vi "Test MPU6050 1.vi"(8 "Error In":errorcluster) -> (0 "error out":errorcluster)   [LabVIEW 2014]
uses:
  <vilib>/LabVIEW Universal Transcriptor/Arduino MPU6050 Library/Arduino MPU6050.lvlib
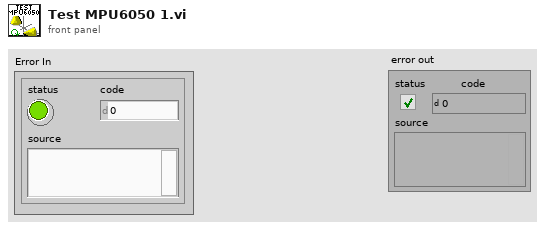
[diagram p1: front panel]
types:
  T1 = enum16{"MPU6050_SCALE_250DPS", "MPU6050_SCALE_500DPS", "MPU6050_SCALE_1000DPS", "MPU6050_SCALE_2000DPS"}
  T2 = enum16{"MPU6050_RANGE_2G", "MPU6050_RANGE_4G", "MPU6050_RANGE_8G", "MPU6050_RANGE_16G"}
  T3 = typedef "Arduino MPU6050.lvlib/Vector.ctl" = cluster{"XAxis":dbl, "YAxis":dbl, "ZAxis":dbl}
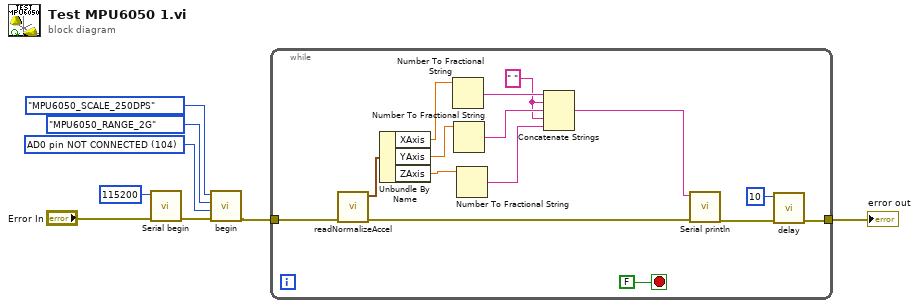
[diagram p0: block diagram]
diagram:
  w3 = u16 104 items=["AD0 pin NOT CONNECTED"=104, "AD0 connect to Vcc"=105] ("address")
  n1 = call <vilib>:"Serial begin.vi"("Error In"="Error In", "speed (Bd)"=115200) -> ("Error Out"=w6:errorcluster)  [unwired: 9 in]
  n2 = call <vilib>:"begin.vi"("Error In"=w6, "address"=w3, "range"=T2."MPU6050_RANGE_2G", "scale"=T1."MPU6050_SCALE_250DPS") -> ("Error Out"=w7:errorcluster)  [unwired: 7 in]
  n3 = while {
    tunnel: w7 -> [w23]
    tunnel: [w17] -> w8
    stop <- FALSE stop-if-true
    w9 = " " ("F-format string")
    n4 = call <vilib>:"readNormalizeAccel.vi"("error in (no error)"=w23) -> ("error out"=w14:errorcluster, "Vector"=w22:T3)  [unwired: 9 in]
    n5 = Unbundle By Name(w22) -> ("XAxis"=w20:dbl, "YAxis"=w19:dbl, "ZAxis"=w18:dbl)
    n6 = Number To Fractional String(number=w20) -> (F-format string=w13:string)  [unwired: 3 in]
    n7 = Number To Fractional String(number=w19) -> (F-format string=w12:string)  [unwired: 3 in]
    n8 = Number To Fractional String(number=w18) -> (F-format string=w11:string)  [unwired: 3 in]
    n9 = Concatenate Strings(w13, w9, w12, w9, w11) -> (w10:string)
    n10 = call <vilib>:"Serial println.vi"("Error In"=w14, "string in"=w10) -> ("Error Out"=w16:errorcluster)  [unwired: 9 in]
    n11 = call <vilib>:"delay.vi"("Error In"=w16, "time (ms)"=10) -> ("Error Out"=w17:errorcluster)  [unwired: 9 in]
  }
  "error out" <- w8
